vi "Simulate Temperature Acquisition - Station 2.vi"() -> (3 "Temperature":dbl)   [LabVIEW 2019]
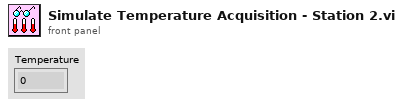
[diagram p1: front panel]
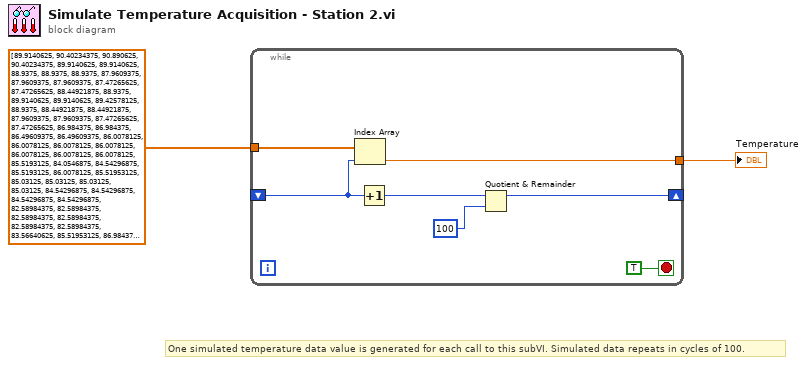
[diagram p0: block diagram]
diagram:
  # "One simulated temperature data value is generated for each call to this subVI. Simulated data repeats in cycles of 100."
  n1 = while {
    tunnel: dbl[] [89.9140625, 90.40234375, 90.890625, 90.40234375, 89.9140625, 89.9140625, 88.9375, 88.9375, 88.9375, 87.9609375, 87.9609375, 87.9609375, 87.47265625, 87.47265625, 88.44921875, 88.9375, 89.9140625, 89.9140625, 89.42578125, 88.9375, 88.44921875, 88.44921875, 87.9609375, 87.9609375, 87.47265625, 87.47265625, 86.984375, 86.984375, 86.49609375, 86.49609375, 86.0078125, 86.0078125, 86.0078125, 86.0078125, 86.0078125, 86.0078125, 86.0078125, 85.5193125, 84.0546875, 84.54296875, 85.5193125, 86.0078125, 85.51953125, 85.03125, 85.03125, 85.03125, 85.03125, 84.54296875, 84.54296875, 84.54296875, 84.54296875, 82.58984375, 82.58984375, 82.58984375, 82.58984375, 82.58984375, 82.58984375, 83.56640625, 85.51953125, 86.984375, 87.47265625, 86.984375, 86.984375, 86.49609375, 86.49609375, 87.9609375, 88.9375, 89.42578125, 89.9140625, 89.9140625, 90.40234375, 89.9140625, 89.42578125, 88.9375, 88.44921875, 88.44921875, 87.9609375, 87.47265625, 86.984375, 86.984375, 86.984375, 86.984375, 86.984375, 86.49609375, 86.49609375, 86.0078125, 86.0078125, 86.0078125, 86.984375, 87.47265625, 87.9609375, 88.44921875, 89.42578125, 89.9140625, 89.9140625, 89.9140625, 89.42578125, 88.9375, 88.44921875, 88.9375] ("array w/ subset deleted") -> [w8]
    tunnel: [w7] -> w2
    shift-right: [w5] -> _
    shift-left: _ -> [w3]
    stop <- TRUE stop-if-true
    n2 = Index Array(array=w8, index=w3) -> (element=w7:dbl)
    n3 = Increment(x=w3) -> (x+1=w4:i32)
    n4 = Quotient & Remainder(x=w4, y=100) -> (x-y*floor(x/y)=w5:i32)  [unwired: 1 out]
  }
  "Temperature" <- w2
